vi "Connect Manager.vi"(6 "Server Certificate File (.crt)":path, 8 "error in (no error)":errorcluster, 9 "VI Reference":refnum<vi>, 10 "Address":string, 11 "CIF_UI in":refnum<class "CIF_UI.lvclass">) -> (0 "error out":errorcluster, 3 "CIF_UI out":refnum<class "CIF_UI.lvclass">)   [LabVIEW 2021, in "CIF_UI.lvclass"]
uses:
  CIF_UI.lvclass
  Typedef/Plugin Connection Map.ctl
  Typedef/Plugin Connections.ctl
  <vilib>/gRPC/LabVIEW gRPC Library/Shared/grpcId.ctl
  CIFPluginManager/CIFPluginManager/gRPC/CIF_Manager_client/RPC Messages/cif_manager_PluginInfo.ctl
  CIFPluginManager/CIFPluginManager/gRPC/CIF_Manager_client/RPC Messages/cif_manager_PluginVersion.ctl
  CIFPluginManager/CIFPluginManager/gRPC/CIF_Manager_client/RPC Messages/cif_plugincore_StatusData.ctl
  CIFPluginManager/CIFPluginManager/gRPC/CIF_Manager_client/RPC Messages/cif_plugincore_StatusData_State.ctl
  CIFPluginManager/CIFPluginManager/gRPC/CIF_Manager_client/RPC Messages/cif_plugincore_TimingStatistics.ctl
  CIFPluginManager/CIFPluginManager/gRPC/CIF_Manager_client/RPC Messages/cif_plugincore_TimingStatsBasic.ctl
  CIFPluginManager/CIFPluginManager/gRPC/CIF_Manager_client/RPC Messages/cif_plugincore_FifoStatistics.ctl
  CIFPluginManager/CIFPluginManager/gRPC/CIF_Manager_client/RPC Messages/cif_plugincore_Error.ctl
  CIFPluginManager/CIFPluginManager/gRPC/CIF_Manager_client/RPC Messages/cif_plugincore_MonitorDoubles.ctl
  CIFPluginManager/CIFPluginManager/gRPC/CIF_Manager_client/RPC Messages/cif_plugincore_MonitorU64.ctl
  CIFPluginManager/CIFPluginManager/gRPC/CIF_Manager_client/RPC Messages/cif_plugincore_MonitorI64.ctl
  CIFCore/Common/Typedef/Errors.ctl
  CIF_UI.lvclass/CIF_UI.ctl
  CIFCore/Common/Utilities/Append Error Location.vi
  CIFPluginManager/CIFPluginManager/gRPC/CIF_Manager_Client_Wrapper/CIFManagerClientWrapper.lvlib
  <vilib>/gRPC/LabVIEW gRPC Library/grpc-lvsupport-release.lvlib
  CIFPluginManager/CIFPluginManager/gRPC/CIF_Manager_client/CIF_Manager_client.lvlib
  CIFCore/Common/CIFCoreCommon.lvlib
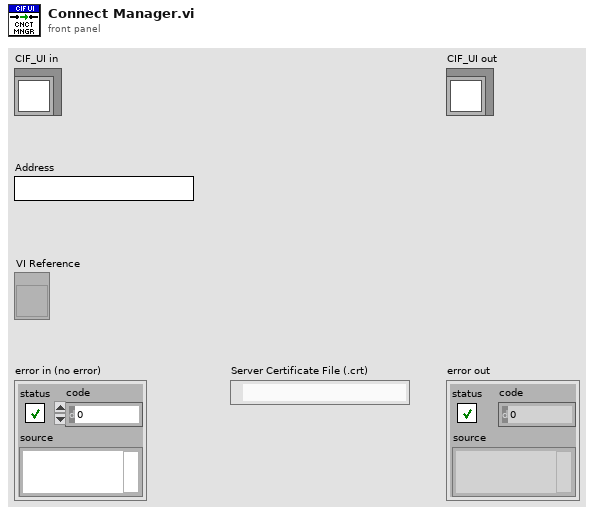
[diagram p1: front panel]
types:
  T1 = typedef "CIFCoreCommon.lvlib/Errors.ctl" = enum16{"Invalid Clock ID", "Long Sleep", "gRPC Server Not Found", "Config Parse", "Timestamp Wrap", "Delayed Execution", "Duplicate Channel", "Missing Channel", "Incorrect Type", "Flatten Error", "Unflatten Data", "Unique Name", "Plugin Not Found", "Plugin Type Not Found", "Plugin Version Not Found", "Manager Not Found", "Numerical Issue", "Time Jump", "Clock ID Match", "Channel Length", "Plugin Connection", "gRPC Server Connection"}
  T2 = typedef "CIF_UI.lvclass/Plugin Connection Map.ctl" = map{string, T3}
  T3 = typedef "CIF_UI.lvclass/Plugin Connections.ctl" = cluster{"gRPC ID":T4, "Plugin info":T5}
  T4 = typedef "grpc-lvsupport-release.lvlib/grpcId.ctl" = u64
  T5 = typedef "CIF_Manager_client.lvlib/cif_manager_PluginInfo.ctl" = cluster{"plugin_name":string, "plugin_type":string, "grpc_port":i32, "plugin_version":T6, "status":T7}
  T6 = typedef "CIF_Manager_client.lvlib/cif_manager_PluginVersion.ctl" = cluster{"major_version":i32, "minor_version":i32, "fix_version":i32, "build_version":i32}
  T7 = typedef "CIF_Manager_client.lvlib/cif_plugincore_StatusData.ctl" = cluster{"state":T8, "timing_statistics":T9, "fifo_statistics":T11, "error":T12, "monitor_doubles":T13, "monitor_u64s":T14, "monitor_i64s":T15}
  T8 = typedef "CIF_Manager_client.lvlib/cif_plugincore_StatusData_State.ctl" = enum32{"NULL", "CREATING", "LISTENING", "RUNNING", "CLEANINGUP", "DESTROYING"}
  T9 = typedef "CIF_Manager_client.lvlib/cif_plugincore_TimingStatistics.ctl" = cluster{"period":T10, "wake_error":T10, "execute":T10, "housekeep":T10, "idle":T10}
  T10 = typedef "CIF_Manager_client.lvlib/cif_plugincore_TimingStatsBasic.ctl" = cluster{"max":i32, "min":i32}
  T11 = typedef "CIF_Manager_client.lvlib/cif_plugincore_FifoStatistics.ctl" = cluster{"from_t0":T10, "from_previous_plugin":T10, "output_error":T10}
  T12 = typedef "CIF_Manager_client.lvlib/cif_plugincore_Error.ctl" = cluster{"status":bool, "code":i32}
  T13 = typedef "CIF_Manager_client.lvlib/cif_plugincore_MonitorDoubles.ctl" = cluster{"double_1":dbl, "double_2":dbl, "double_3":dbl, "double_4":dbl}
  T14 = typedef "CIF_Manager_client.lvlib/cif_plugincore_MonitorU64.ctl" = cluster{"u64_1":u64, "u64_2":u64, "u64_3":u64, "u64_4":u64}
  T15 = typedef "CIF_Manager_client.lvlib/cif_plugincore_MonitorI64.ctl" = cluster{"i64_1":i64, "i64_2":i64, "i64_3":i64, "i64_4":i64}
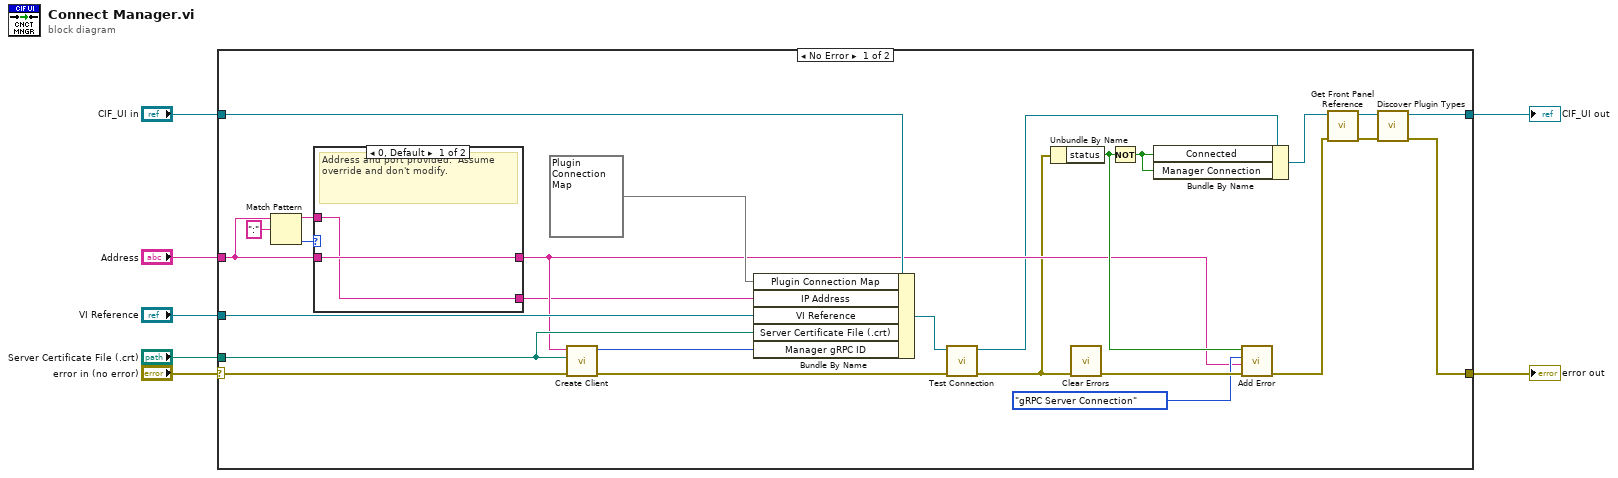
[diagram p0: block diagram]
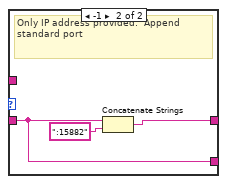
[diagram p2: hidden frame]
diagram:
  n1 = case shown="No Error" "error in (no error)" {
    selector: "error in (no error)" -> [w31 w40]
    tunnel: [w9 w40] -> w6
    tunnel: [w8 w39] -> w4
    tunnel: "CIF_UI in" -> [w32 w39]
    tunnel: "Address" -> [w28 _]
    tunnel: "VI Reference" -> [w33 _]
    tunnel: "Server Certificate File (.crt)" -> [w27 _]
    frame No Error {
      n2 = Match Pattern(string=w28, regular expression=":") -> (before substring=w13:string, offset past match=w30:i32)  [unwired: 1 in, 2 out]
      n3 = case shown="0, Default" w30 {
        tunnel: w28 -> [w35 w36]
        tunnel: [w35 w38] -> w19
        tunnel: [w34 w36] -> w14
        tunnel: w13 -> [w34 _]
        frame 0, Default {
          # "Address and port provided.  Assume override and don't modify."
        }
        frame -1 {
          # "Only IP address provided.  Append standard port"
          n4 = Concatenate Strings(w36, ":15882" ("string")) -> (w38:string)
        }
      }
      n5 = call "Create Client.vi"("error in"=w31, "Server Certificate File (.crt)"=w27, "address"=w19) -> ("error out"=w17:errorcluster, "gRPC ID Out"=w25:T4)  [unwired: 7 in]
      n6 = Bundle By Name(cluster=w32, "Plugin Connection Map"=T2 {}, "IP Address"=w14, "VI Reference"=w33, "Server Certificate File (.crt)"=w27, "Manager gRPC ID"=w25) -> (w18:refnum<class "CIF_UI.lvclass">)
      n7 = call "Test Connection.vi"("error in (no error)"=w17, "CIF_UI in"=w18) -> ("error out"=w16:errorcluster, "CIF_UI out"=w15:refnum<class "CIF_UI.lvclass">)  [unwired: 8 in]
      n8 = Unbundle By Name(w16) -> ("status"=w21:bool)
      n9 = call <vilib>:"Clear Errors.vi"("error in (no error)"=w16) -> ("error out"=w23:errorcluster)  [unwired: 5 in, 1 out]
      n10 = Not(x=w21) -> (.not. x?=w12:bool)
      n11 = Bundle By Name(cluster=w15, "Connected"=w12, "Manager Connection"=w12) -> (w24:refnum<class "CIF_UI.lvclass">)
      n12 = call "Add Error.vi"("error in (no error)"=w23, "String to Append"=w19, "Error"=Errors."gRPC Server Connection", "Insert Error"=w21) -> ("error out"=w22:errorcluster)  [unwired: 7 in]
      n13 = call "Get Front Panel Reference.vi"("error in (no error)"=w22, "CIF_UI in"=w24) -> ("error out"=w10:errorcluster, "CIF_UI out"=w11:refnum<class "CIF_UI.lvclass">)  [unwired: 8 in]
      n14 = call "Discover Plugin Types.vi"("error in (no error)"=w10, "CIF_UI in"=w11) -> ("error out"=w9:errorcluster, "CIF_UI out"=w8:refnum<class "CIF_UI.lvclass">)  [unwired: 8 in]
    }
    frame Error {
    }
  }
  "error out" <- w6
  "CIF_UI out" <- w4
